vi "Read CSV File (UTF-16).vi"(7 "delimiter (,) *ASCII":string=",", 8 "error in (no error)":errorcluster, 11 "file path in":path) -> (0 "error out":errorcluster, 2 "2-D array *UTF-16":string[][](array[string]), 3 "file path out":path)   [LabVIEW 2013, in "SET_Robust CSV (UTF-16).lvlib"]
doc: "Reads a CSV (Character Separated Values) spreadsheet file to a 2D array of strings.\nThe CSV spreadsheet is assumed to be ANSI encoded and formatted in accordance with RFC-4180 (see http://tools.ietf.org/html/rfc4180). \nAll EOLs (CR, LF or CR+LF) will be converted to LF and all escaped double quotes will be un-escaped in the output array.\n\nRev 0.0 2014-02-20 Ryan Porter\nFirst Draft"
uses:
  SET_Robust CSV (UTF-16).lvlib
panel:
  # "Read CSV File.vi\n\nReads a CSV (Character Separated Values) spreadsheet file to a 2D array of strings.\nThe CSV spreadsheet is assumed to be UTF-16 LE encoded and formatted in accordance with RFC-4180 (see http://tools.ietf.org/html/rfc4180). \nAll EOLs (CR, LF or CR+LF) will be converted to LF and all escaped double quotes will be un-escaped in the output array."
  # "License: BSD (2-Clause) - http://opensource.org/licenses/BSD-2-Clause \n\nCopyright (c) 2014, Ryan Porter\nAll rights reserved."
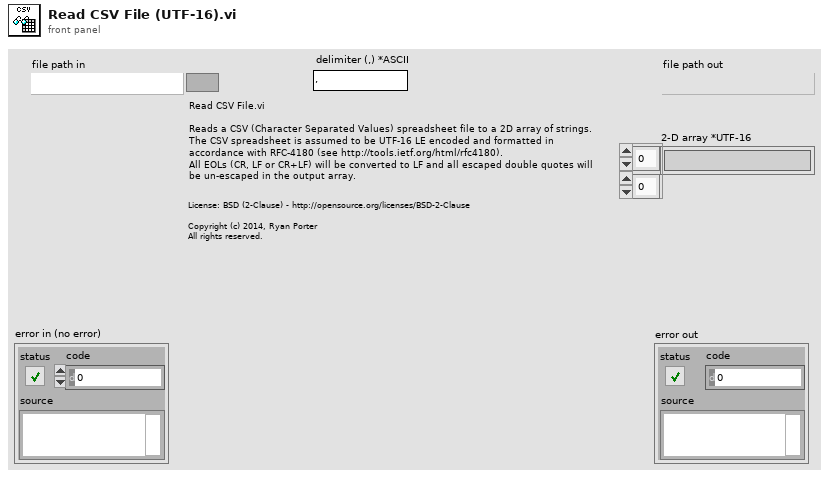
[diagram p1: front panel]
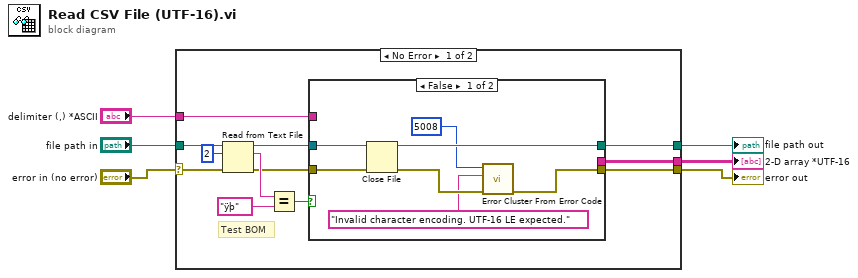
[diagram p0: block diagram]
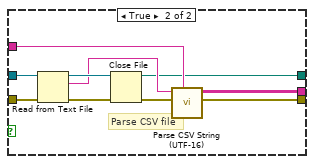
[diagram p2: hidden frame]
diagram:
  n1 = case shown="No Error" "error in (no error)" {
    selector: "error in (no error)" -> [w12 w36]
    tunnel: "file path in" -> [w13 w37]
    tunnel: [w15 _] -> w2
    tunnel: "delimiter (,) *ASCII" -> [w18 _]
    tunnel: [w17 w37] -> w3
    tunnel: [w16 w36] -> w1
    frame No Error {
      # "Test BOM"
      n2 = Read from Text File(file (use dialog)=w13, count=2, error in=w12) -> (refnum out=w8:refnum<file>, text=w10:string, error out=w9:errorcluster)  [unwired: 1 in, 1 out]
      n3 = Equal?(x=w10, y="ÿþ") -> (x = y?=w7:bool)
      n4 = case shown="False" w7 {
        tunnel: w18 -> [_ w32]
        tunnel: [w25 w31] -> w17
        tunnel: [w21 w29] -> w16
        tunnel: [_ w28] -> w15
        tunnel: w9 -> [w23 w27]
        tunnel: w8 -> [w24 w26]
        frame False {
          n5 = Close File(refnum=w24, error in=w23) -> (path=w25:path, error out=w22:errorcluster)
          n6 = call <vilib>:"Error Cluster From Error Code.vi"("error in (no error)"=w22, "error message (\"\")"="Invalid character encoding. UTF-16 LE expected." ("error message (\"\")"), "error code (0)"=5008) -> ("error out"=w21:errorcluster)  [unwired: 6 in]
        }
        frame True {
          # "Parse CSV file"
          n7 = Read from Text File(file (use dialog)=w26, error in=w27) -> (refnum out=w35:refnum<file>, text=w33:string, error out=w34:errorcluster)  [unwired: 2 in, 1 out]
          n8 = Close File(refnum=w35, error in=w34) -> (path=w31:path, error out=w30:errorcluster)
          n9 = call "Parse CSV String (UTF-16).vi"("delimiter (,) *ASCII"=w32, "error in"=w30, "CSV string *UTF-16"=w33) -> ("error out"=w29:errorcluster, "2-D array *UTF-16"=w28:string[][])  [unwired: 7 in]
        }
      }
    }
    frame Error {
    }
  }
  "2-D array *UTF-16" <- w2
  "error out" <- w1
  "file path out" <- w3
